vi "tcp_load.vi"(0 "freq_array_in":dbl[](array[numeric]), 1 "freq_range":cluster{"start_freq":string, "stop_freq":string}, 2 "data_in":cluster{"s11_s21":string, "trace_data":string}, 3 "new_data_available":bool, 5 "data_array_in":dbl[][](array[numeric]), 9 "freq_available_in":bool, 11 "data_available_in":T1) -> (4 "freq_array_out":dbl[](array[numeric]), 6 "data_array_out":dbl[][](array[numeric]), 10 "freq_available_out":bool, 15 "data_available_out":T1)   [LabVIEW 2025]
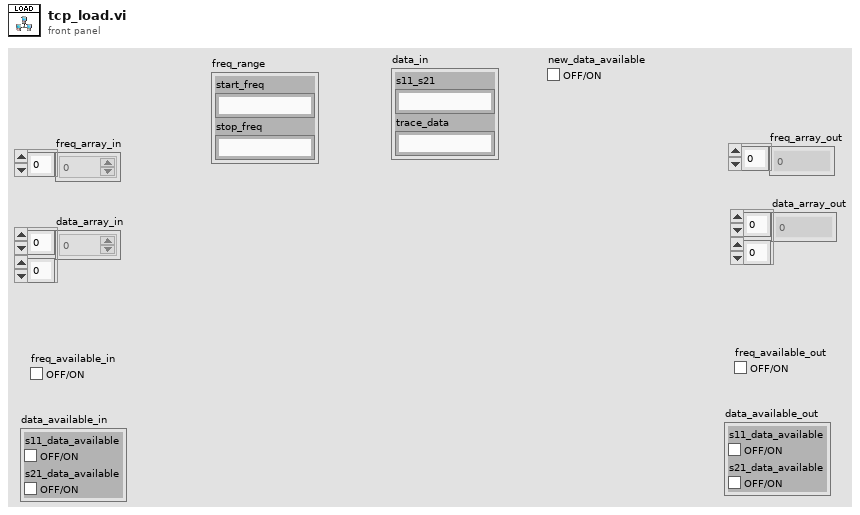
[diagram p1: front panel]
types:
  T1 = cluster{"s11_data_available":bool, "s21_data_available":bool}
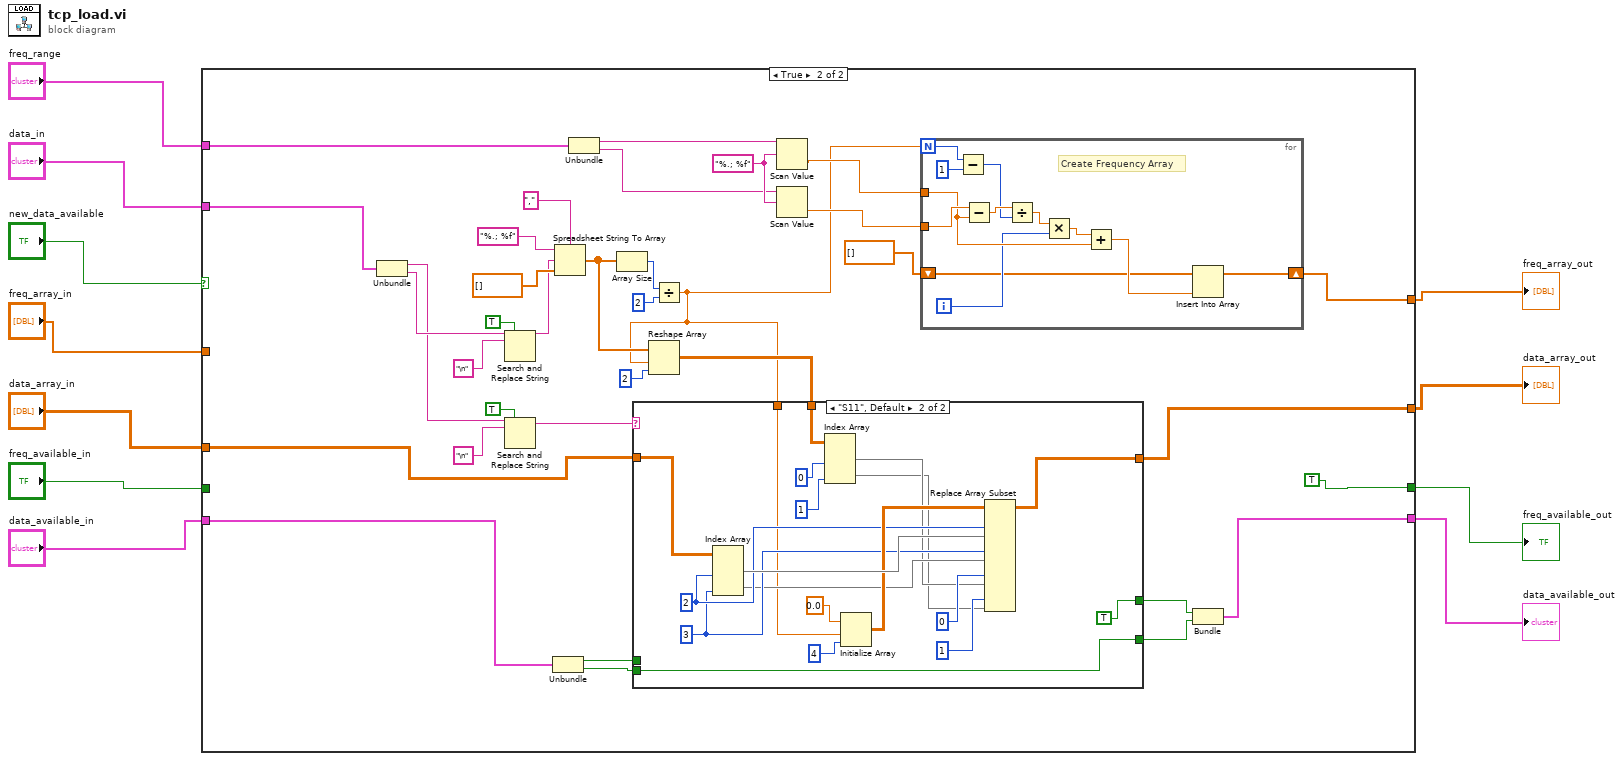
[diagram p0: block diagram]
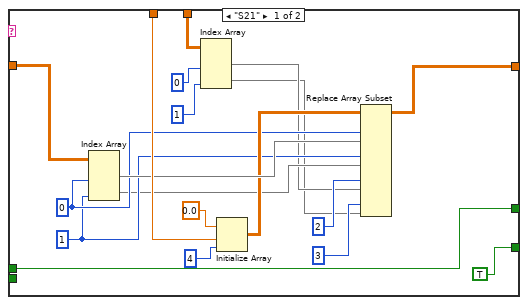
[diagram p3: hidden frame]
diagram:
  n1 = case shown="True" "new_data_available" {
    tunnel: [w12 w48] -> w3
    tunnel: [w15 TRUE ("freq_available_in")] -> w10
    tunnel: "freq_available_in" -> [w15 _]
    tunnel: "data_array_in" -> [w14 w50]
    tunnel: [w14 w47] -> w8
    tunnel: [w13 w46] -> w7
    tunnel: "freq_array_in" -> [w13 _]
    tunnel: "freq_range" -> [_ w45]
    tunnel: "data_in" -> [_ w44]
    tunnel: "data_available_in" -> [w12 w43]
    frame False {
    }
    frame True {
      w31 = "%.; %f" ("format string")
      n2 = Unbundle(w44) -> ("s11_s21"=w18:string, "trace_data"=w26:string)
      n3 = Search and Replace String(replace all?=TRUE ("replace all? (F)"), input string=w26, search string="\n") -> (result string=w37:string)  [unwired: 5 in, 3 out]
      n4 = Search and Replace String(replace all?=TRUE ("replace all? (F)"), input string=w18, search string="\n") -> (result string=w17:string)  [unwired: 5 in, 3 out]
      n5 = Unbundle(w43) -> ("s11_data_available"=w22:bool, "s21_data_available"=w21:bool)
      n6 = Spreadsheet String To Array(delimiter (Tab)=",", format string="%.; %f", spreadsheet string=w37, array type (2D Dbl)=dbl[] []) -> (array=w33:dbl[])
      n7 = Unbundle(w45) -> ("start_freq"=w30:string, "stop_freq"=w29:string)
      n8 = Array Size(array=w33) -> (size(s)=w35:i32)
      n9 = Divide(x=w35, y=2) -> (x/y=w16:dbl)
      n10 = Reshape Array(w33, w16, 2 ("dimension size")) -> (w25:dbl[][])
      n11 = case shown="\"S11\", Default" w17 {
        tunnel: w25 -> [w58 w72]
        tunnel: [w51 w70] -> w47
        tunnel: [w68 TRUE ("s11_data_available")] -> w24
        tunnel: [TRUE ("s21_data_available") w87] -> w23
        tunnel: w22 -> [w68 _]
        tunnel: w21 -> [_ w87]
        tunnel: w16 -> [w66 w71]
        tunnel: w50 -> [w64 w73]
        frame "S21" {
          w60 = 1 ("index (col)")
          w61 = 0 ("index (col)")
          n12 = Index Array(array=w64, index (col) #1=w61, index (col) #2=w60) -> (element #1=w63:dbl[], element #2=w59:dbl[])  [unwired: 2 in]
          n13 = Index Array(array=w58, index (col) #1=0 ("index (col)"), index (col) #2=1 ("index (col)")) -> (element #1=w53:dbl[], element #2=w52:dbl[])  [unwired: 2 in]
          n14 = Initialize Array(0.0 ("element"), w66, 4 ("dimension size")) -> (w62:dbl[][])
          n15 = Replace Array Subset(array=w62, new element #1=w63, index (col) #1=w61, new element #2=w59, index (col) #2=w60, new element #3=w53, index (col) #3=2 ("index (col)"), new element #4=w52, index (col) #4=3 ("index (col)")) -> (w51:dbl[][])  [unwired: 4 in]
        }
        frame "S11", Default {
          w81 = 3 ("index (col)")
          w82 = 2 ("index (col)")
          n16 = Index Array(array=w73, index (col) #1=w82, index (col) #2=w81) -> (element #1=w84:dbl[], element #2=w80:dbl[])  [unwired: 2 in]
          n17 = Index Array(array=w72, index (col) #1=0 ("index (col)"), index (col) #2=1 ("index (col)")) -> (element #1=w75:dbl[], element #2=w74:dbl[])  [unwired: 2 in]
          n18 = Initialize Array(0.0 ("element"), w71, 4 ("dimension size")) -> (w83:dbl[][])
          n19 = Replace Array Subset(array=w83, new element #1=w84, index (col) #1=w82, new element #2=w80, index (col) #2=w81, new element #3=w75, index (col) #3=0 ("index (col)"), new element #4=w74, index (col) #4=1 ("index (col)")) -> (w70:dbl[][])  [unwired: 4 in]
        }
      }
      n20 = Scan Value(string=w30, format string=w31) -> (value=w28:dbl)  [unwired: 1 in, 1 out]
      n21 = Scan Value(string=w29, format string=w31) -> (value=w27:dbl)  [unwired: 1 in, 1 out]
      n22 = for {
        N: w16 -> [w93]
        shift-right: [w95] -> w46
        shift-left: dbl[] [] -> [w89]
        tunnel: w28 -> [w96]
        tunnel: w27 -> [w100]
        i -> [w90]
        # "Create Frequency Array"
        n23 = Subtract(x=w93, y=1) -> (x-y=w92:i32)
        n24 = Subtract(x=w100, y=w96) -> (x-y=w99:dbl)
        n25 = Divide(x=w99, y=w92) -> (x/y=w98:dbl)
        n26 = Multiply(x=w98, y=w90) -> (x*y=w97:dbl)
        n27 = Add(x=w97, y=w96) -> (x+y=w94:dbl)
        n28 = Insert Into Array(array=w89, new element=w94) -> (w95:dbl[])  [unwired: 1 in]
      }
      n29 = Bundle("s11_data_available"=w24, "s21_data_available"=w23) -> (w48:T1)  [unwired: 1 in]
    }
  }
  "freq_available_out" <- w10
  "data_array_out" <- w8
  "freq_array_out" <- w7
  "data_available_out" <- w3
